vi "CreateEvents.vi"(8 "error in (no error)":errorcluster, 11 "JQMHCore in":refnum<class "Module.lvclass">) -> (0 "error out":errorcluster, 3 "JQMHCore out":refnum<class "Module.lvclass">)   [LabVIEW 2024, in "Module.lvclass"]
uses:
  Module.lvclass
  Module.lvclass/Module.ctl
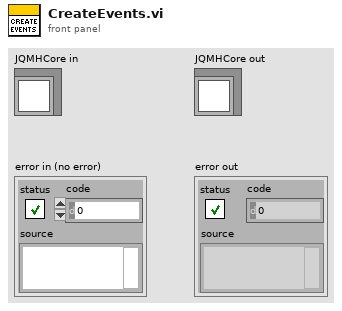
[diagram p1: front panel]
types:
  T1 = typedef "Module.lvclass/StandardRequests.ctl" = cluster{"Initialise":refnum<user-event>, "Stop Module":refnum<user-event>, "ShowFP":refnum<user-event>, "Hide Front Panel":refnum<user-event>, "Show Block Diagram":refnum<user-event>, "Hide Block Diagram":refnum<user-event>}
  T2 = typedef "Module.lvclass/StandardBroadcasts.ctl" = cluster{"Died":refnum<user-event>, "Started":refnum<user-event>}
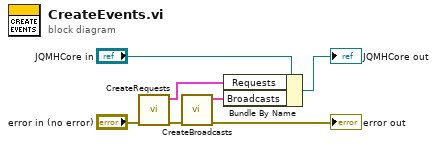
[diagram p0: block diagram]
diagram:
  n1 = call "CreateRequests.vi"("error in (no error)"="error in (no error)") -> ("error out"=w3:errorcluster, "StandardRequests"=w4:T1)  [unwired: 9 in]
  n2 = call "CreateBroadcasts.vi"("error in (no error)"=w3) -> ("error out"=→"error out":errorcluster, "StandardBroadcasts"=w1:T2)  [unwired: 9 in]
  n3 = Bundle By Name(cluster="JQMHCore in", "Requests"=w4, "Broadcasts"=w1) -> (→"JQMHCore out":refnum<class "Module.lvclass">)
